vi "Control Labels.vi"(11 "MetaDataObj.lvclass":refnum<class "MetaDataObj.lvclass">) -> (2 "localized control labels":string[](array[string]), 3 "DNL_unlocalized control labels":string[](array[string]), 4 "DNL_unlocalized string constant labels":string[](array[string]), 6 "localized string constant values":string[](array[string]))   [LabVIEW 2016, in "MetaDataObj.lvclass"]
doc: "Override this VI to supply the control label localizations. The first array is the label text as it appears in your unmodified template VIs. The second array is the label text as it should appear in the user's instantiated VIs. You may dynamically generate the second array based on user values obtained through the New Project Wizard and your spec page VI."
uses:
  <resource>/dialog/NewProjectWizard/MetaDataObj/MetaDataObj.lvclass
  <resource>/dialog/NewProjectWizard/MetaDataObj/MetaDataObj.lvclass/MetaDataObj.ctl
  <resource>/dialog/NewProjectWizard/MetaDataObj/Accessors/Read Label Localizations.vi
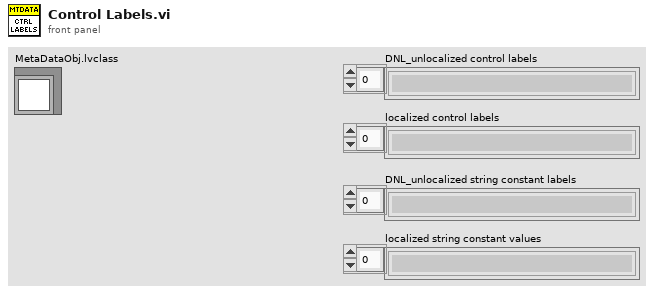
[diagram p1: front panel]
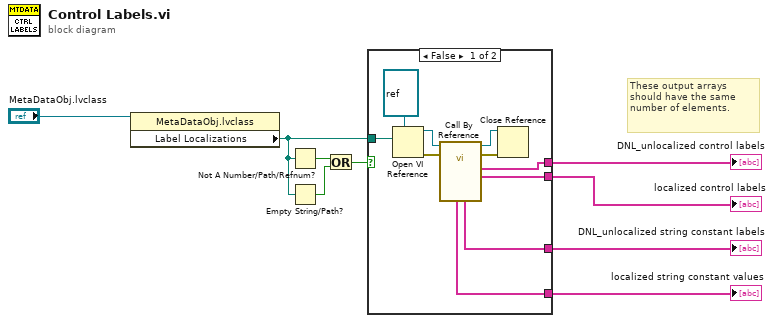
[diagram p0: block diagram]
diagram:
  # "These output arrays should have the same number of elements."
  n1 = property class="MetaDataObj.lvclass"(reference="MetaDataObj.lvclass") -> ("Label Localizations"=w5:path)  [unwired: 1 in, 2 out]
  n2 = Not A Number/Path/Refnum?(number/path/refnum=w5) -> (NaN/Path/Refnum?=w8:bool)
  n3 = Empty String/Path?(string/path=w5) -> (empty?=w7:bool)
  n4 = Or(x=w8, y=w7) -> (x .or. y?=w6:bool)
  n5 = case shown="False" w6 {
    tunnel: w5 -> [w19 _]
    tunnel: [w13 _] -> w4
    tunnel: [w12 _] -> w3
    tunnel: [w11 _] -> w2
    tunnel: [w10 _] -> w1
    frame False {
      n6 = Open VI Reference(type specifier VI Refnum (for type only)=refnum<vi> refnum, vi path=w19) -> (vi reference=w17:refnum<vi>, error out=w15:errorcluster)  [unwired: 4 in]
      n7 = call-by-ref "?"(reference=w17, error in=w15) -> (reference out=w16:refnum<vi>, error out=w14:errorcluster, "localized control labels"=w12:string[], "DNL_unlocalized control labels"=w13:string[], "DNL_unlocalized string constant labels"=w11:string[], "localized string constant values"=w10:string[])  [unwired: 8 in]
      n8 = Close Reference(reference=w16, error in (no error)=w14) -> ()  [unwired: 1 out]
    }
    frame True {
    }
  }
  "localized control labels" <- w3
  "DNL_unlocalized control labels" <- w4
  "localized string constant values" <- w1
  "DNL_unlocalized string constant labels" <- w2
